vi "Get Velocity Data.vi"(8 "error in (no error)":errorcluster, 10 "Complete NMEA Sentences":string[](array[string]), 11 "VISA resource name":refnum<visa-resource-name>) -> (0 "error out":errorcluster, 1 "Velocity Data":cluster{"Bearing":dbl, "Speed":dbl}[](array[cluster]), 2 "Complete NMEA Sentences (Copy)":string[](array[string]), 3 "VISA resource name out":refnum<visa-resource-name>)   [LabVIEW 2009]
doc: "Parses out the velocity data from all of the sentences that Read Raw.vi outputs, and passes through a complete copy of those sentences. Can be used in conjunction with other advanced \"Get\" VIs. See u-blox 5 Series Acquire and Chart GPS Advanced.vi for an example of how to use this VI.\n\nNote that the VISA Resource is not required, since this VI is a helper that does not actually interact with the device. The VISA Resource can be used, however, to clarify programming and maintain uniformity."
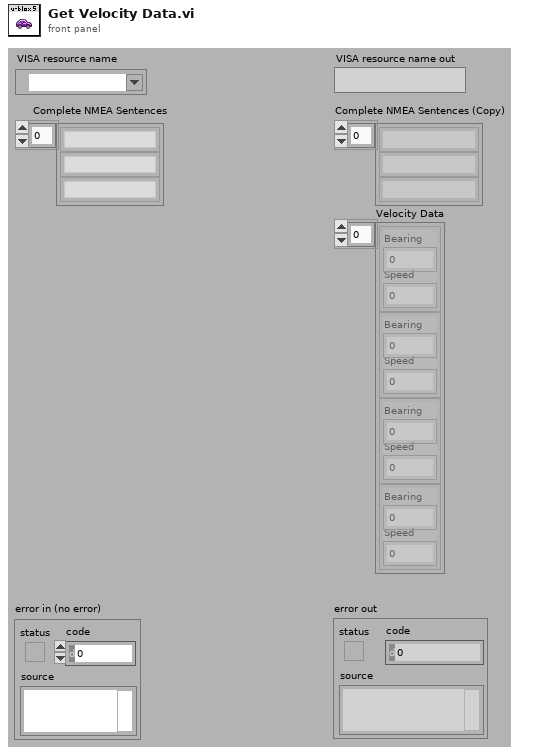
[diagram p1: front panel]
types:
  T1 = typedef "VTG Data.ctl" = cluster{"true track made good":cluster{"included?":bool, "true track made good (deg)":dbl}, "magnetic track made good":cluster{"included?":bool, "magnetic track made good (deg)":dbl}, "ground speed (knots)":cluster{"included?":bool, "speed (knots)":dbl}, "ground speed (km/h)":cluster{"included?":bool, "speed (km/h)":dbl}, "type of fix":cluster{"included?":bool, "mode":u16}}
  T2 = typedef "RMC Data.ctl" = cluster{"time of fix":cluster{"included?":bool, "time":timestamp}, "status":cluster{"included?":bool, "value":u16}, "latitude":cluster{"included?":bool, "latitude (deg)":dbl}, "longitude":cluster{"included?":bool, "longitude (deg)":dbl}, "ground speed":cluster{"included?":bool, "speed (knots)":dbl}, "true track angle":cluster{"included?":bool, "angle (deg)":dbl}, "magnetic variation":cluster{"included?":bool, "variation (deg)":dbl}, "type of fix":cluster{"included?":bool, "mode":u16}}
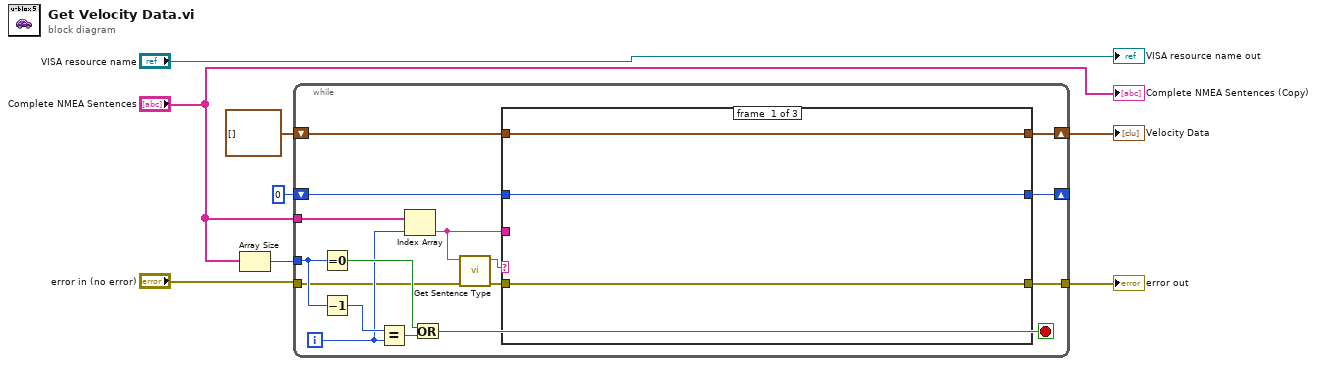
[diagram p0: block diagram]
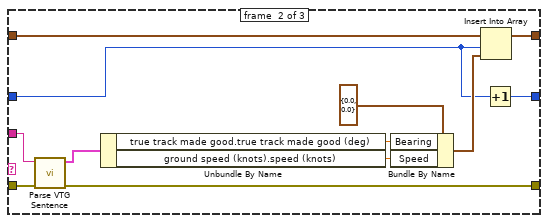
[diagram p2: hidden frame]
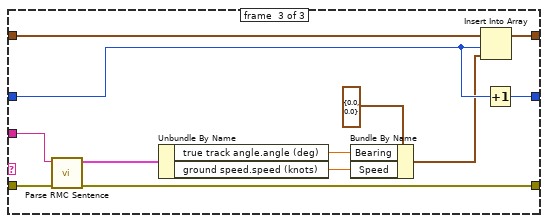
[diagram p3: hidden frame]
diagram:
  n1 = Array Size(array="Complete NMEA Sentences") -> (size(s)=w8:i32)
  n2 = while {
    tunnel: "Complete NMEA Sentences" -> [w24]
    shift-right: [w22] -> w1
    shift-left: cluster{"Bearing":dbl, "Speed":dbl}[] [] -> [w21]
    tunnel: w8 -> [w17]
    tunnel: "error in (no error)" -> [w12]
    tunnel: [w23] -> w6
    shift-right: [w19] -> _
    shift-left: 0 -> [w20]
    i -> [w13]
    stop <- w15 stop-if-true
    n3 = Equal To 0?(x=w17) -> (x = 0?=w16:bool)
    n4 = Decrement(x=w17) -> (x-1=w18:i32)
    n5 = Equal?(x=w18, y=w13) -> (x = y?=w14:bool)
    n6 = Index Array(array=w24, index=w13) -> (element=w9:string)
    n7 = Or(x=w16, y=w14) -> (x .or. y?=w15:bool)
    n8 = call "Get Sentence Type.vi"("error in (no error)"=w12, "sentence"=w9) -> ("error out"=w11:errorcluster, "sentence type"=w10:string)  [unwired: 7 in, 1 out]
    n9 = case shown="\"\", Default" w10 {
      tunnel: w9 -> [_ w29 w41]
      tunnel: w11 -> [w27 w30 w42]
      tunnel: [w27 w31 w43] -> w23
      tunnel: [w26 w33 w45] -> w22
      tunnel: w21 -> [w26 w34 w46]
      tunnel: w20 -> [w25 w32 w50]
      tunnel: [w25 w39 w51] -> w19
      frame #0 {
      }
      frame #1 {
        n10 = call "Parse VTG Sentence.vi"("error in (no error)"=w30, "VTG sentence"=w29) -> ("error out"=w31:errorcluster, "VTG  data"=w28:T1)  [unwired: 8 in]
        n11 = Unbundle By Name(w28) -> ("true track made good.true track made good (deg)"=w37:dbl, "ground speed (knots).speed (knots)"=w38:dbl)
        n12 = Bundle By Name(cluster=cluster{"Bearing":dbl, "Speed":dbl} {"Bearing"=0.0, "Speed"=0.0}, "Bearing"=w37, "Speed"=w38) -> (w35:cluster{"Bearing":dbl, "Speed":dbl})
        n13 = Insert Into Array(array=w34, index=w32, new element=w35) -> (w33:cluster{"Bearing":dbl, "Speed":dbl}[])
        n14 = Increment(x=w32) -> (x+1=w39:i32)
      }
      frame #2 {
        n15 = call "Parse RMC Sentence.vi"("error in (no error)"=w42, "RMC sentence"=w41) -> ("error out"=w43:errorcluster, "RMC data"=w40:T2)  [unwired: 8 in]
        n16 = Unbundle By Name(w40) -> ("true track angle.angle (deg)"=w48:dbl, "ground speed.speed (knots)"=w49:dbl)
        n17 = Bundle By Name(cluster=cluster{"Bearing":dbl, "Speed":dbl} {"Bearing"=0.0, "Speed"=0.0}, "Bearing"=w48, "Speed"=w49) -> (w47:cluster{"Bearing":dbl, "Speed":dbl})
        n18 = Insert Into Array(array=w46, index=w50, new element=w47) -> (w45:cluster{"Bearing":dbl, "Speed":dbl}[])
        n19 = Increment(x=w50) -> (x+1=w51:i32)
      }
    }
  }
  "error out" <- w6
  "Velocity Data" <- w1
  "VISA resource name out" <- "VISA resource name"
  "Complete NMEA Sentences (Copy)" <- "Complete NMEA Sentences"
